vi "Get Log Settings.vi"(0 "Log Ref in":T2 format="%.0x", 7 "RT Data in":T1={"Device Ref"=18446744073709551615, "Waveforms"=[], "Channels"={"Command Chan Refs"=[], "Command Data Refs"=[], "Command Values"=[], "Status Chan Refs"=[], "Status Data Refs"=[], "Status Values"=[], "System Time"={"System Time"=timestamp(0 s since 1904-01-01), "Data Reference"=0, "Absolute Time Channel Data Ref"=0, "Get Date-Time Channel Data Ref"=0}, "Trigger Chan Refs"=[], "Trigger Data Refs"=[], "Trigger Values"=[]}, "Waveform Logs"=[], "Communication"={"Async Status"=refnum, "Wfm Comm Properties"={"WPL"={"Custom Queue Size"=1, "Use Custom Queue Size?"=FALSE}}, "Shutdown Event"=refnum, "Trigger Event"=refnum, "New File Event"=refnum, "Log Queues"=[], "Async VI Ref"=refnum}, "error"={"status"=FALSE, "code"=0, "source"=""}} {"Device Ref" format="%.0x"; "Channels"."Trigger Data Refs"."Data Reference" format="%.0x"; "Channels"."Trigger Chan Refs" format="%.0x"; "Channels"."System Time"."Get Date-Time Channel Data Ref" format="%.0x"; "Channels"."System Time"."Absolute Time Channel Data Ref" format="%.0x"; "Channels"."System Time"."Channel Data Reference" format="%.0x"; "Channels"."Status Data Refs"."Data Reference" format="%.0x"; "Channels"."Command Data Refs"."Data Reference" format="%.0x"; "Channels"."Status Chan Refs" format="%.0x"; "Channels"."Command Chan Refs" format="%.0x"; "Waveforms"."Waveform Ref in" format="%.0x"; "Waveform Logs"."Node ID" format="%.0x"; "Waveform Logs"."TDMS Error Code"."Data Ref" format="%.0x"; "Waveform Logs"."Missed Samples"."Data Ref" format="%.0x"; "Waveform Logs"."File Status"."Data Ref" format="%.0x"; "Waveform Logs"."Start New File"."Data Ref" format="%.0x"; "Waveform Logs"."Logging Enabled"."Data Ref" format="%.0x"; "Waveform Logs"."Stop Trigger"."Node Data Ref" format="%.0x"; "Waveform Logs"."Stop Trigger"."Node ID" format="%.0x"; "Waveform Logs"."Start Trigger"."Node Data Ref" format="%.0x"; "Waveform Logs"."Start Trigger"."Node ID" format="%.0x"}, 11 "Log Index in":i32) -> (8 "RT Data out":T1={"Device Ref"=18446744073709551615, "Waveforms"=[], "Channels"={"Command Chan Refs"=[], "Command Data Refs"=[], "Command Values"=[], "Status Chan Refs"=[], "Status Data Refs"=[], "Status Values"=[], "System Time"={"System Time"=timestamp(0 s since 1904-01-01), "Data Reference"=0, "Absolute Time Channel Data Ref"=0, "Get Date-Time Channel Data Ref"=0}, "Trigger Chan Refs"=[], "Trigger Data Refs"=[], "Trigger Values"=[]}, "Waveform Logs"=[], "Communication"={"Async Status"=refnum, "Wfm Comm Properties"={"WPL"={"Custom Queue Size"=1, "Use Custom Queue Size?"=FALSE}}, "Shutdown Event"=refnum, "Trigger Event"=refnum, "New File Event"=refnum, "Log Queues"=[], "Async VI Ref"=refnum}, "error"={"status"=FALSE, "code"=0, "source"=""}} {"Device Ref" format="%.0x"; "Channels"."Trigger Data Refs"."Data Reference" format="%.0x"; "Channels"."Trigger Chan Refs" format="%.0x"; "Channels"."System Time"."Get Date-Time Channel Data Ref" format="%.0x"; "Channels"."System Time"."Absolute Time Channel Data Ref" format="%.0x"; "Channels"."System Time"."Channel Data Reference" format="%.0x"; "Channels"."Status Data Refs"."Data Reference" format="%.0x"; "Channels"."Command Data Refs"."Data Reference" format="%.0x"; "Channels"."Status Chan Refs" format="%.0x"; "Channels"."Command Chan Refs" format="%.0x"; "Waveforms"."Waveform Ref in" format="%.0x"; "Waveform Logs"."Node ID" format="%.0x"; "Waveform Logs"."TDMS Error Code"."Data Ref" format="%.0x"; "Waveform Logs"."Missed Samples"."Data Ref" format="%.0x"; "Waveform Logs"."File Status"."Data Ref" format="%.0x"; "Waveform Logs"."Start New File"."Data Ref" format="%.0x"; "Waveform Logs"."Logging Enabled"."Data Ref" format="%.0x"; "Waveform Logs"."Stop Trigger"."Node Data Ref" format="%.0x"; "Waveform Logs"."Stop Trigger"."Node ID" format="%.0x"; "Waveform Logs"."Start Trigger"."Node Data Ref" format="%.0x"; "Waveform Logs"."Start Trigger"."Node ID" format="%.0x"}, 15 "Log Index out":i32)   [LabVIEW 2015, in "Waveform Data Logger Engine.lvlib"]
uses:
  Waveform Data Logger Engine.lvlib
  <vilib>/NI Veristand/Custom Device API/Custom Device Item Ref.ctl
  Types/RT Data.ctl
  Types/Inline Waveform Info.ctl
  <vilib>/NI Veristand/Custom Device API/Waveform Data Reference.ctl
  Classes/Waveforms/Waveform Receive/Associated Log.ctl
  <vilib>/NI Veristand/Custom Device API/Custom Device Waveform DataType.ctl
  Types/Channels.ctl
  <vilib>/NI Veristand/Custom Device API/Block Data Reference.ctl
  <vilib>/NI Veristand/Custom Device API/Data Reference.ctl
  Types/System Time.ctl
  Types/Inline Waveform Log Info.ctl
  Classes/Log File Specifications/Waveform TDMS Log File Specification/Waveform TDMS Log File Specification.lvclass
  Classes/Triggers/Trigger/Trigger.lvclass
  Types/Inline Log Waveform.ctl
  Types/Trigger Settings.ctl
  Types/Log Status.ctl
  Types/Channel.ctl
  Types/Communication.ctl
  Types/Async Status.ctl
  Types/Async State.ctl
  <vilib>/NI Veristand/Custom Device Waveform API/Communication Properties.ctl
  Types/Trigger Event Data.ctl
  Types/Trigger Received.ctl
  Types/New File Event Data.ctl
  Types/Log Queues.ctl
  Shared/Globals/Property Strings.vi
  Shared/Globals/Global GUIDs.vi
  <vilib>/NI Veristand/Custom Device API/Get Item Property (Boolean).vi
  <vilib>/NI Veristand/Custom Device API/Get Item Property (U16).vi
  <vilib>/NI Veristand/Custom Device API/Get Item Property (Double).vi
  <vilib>/NI Veristand/Custom Device API/Custom Device API.lvlib
  Shared/Waveform Data Logger Shared.lvlib
  Classes/Waveforms/Waveform Receive/Waveform Receive.lvclass
  <vilib>/NI Veristand/Custom Device Waveform API/NI_VS Custom Device Waveform API.lvlib
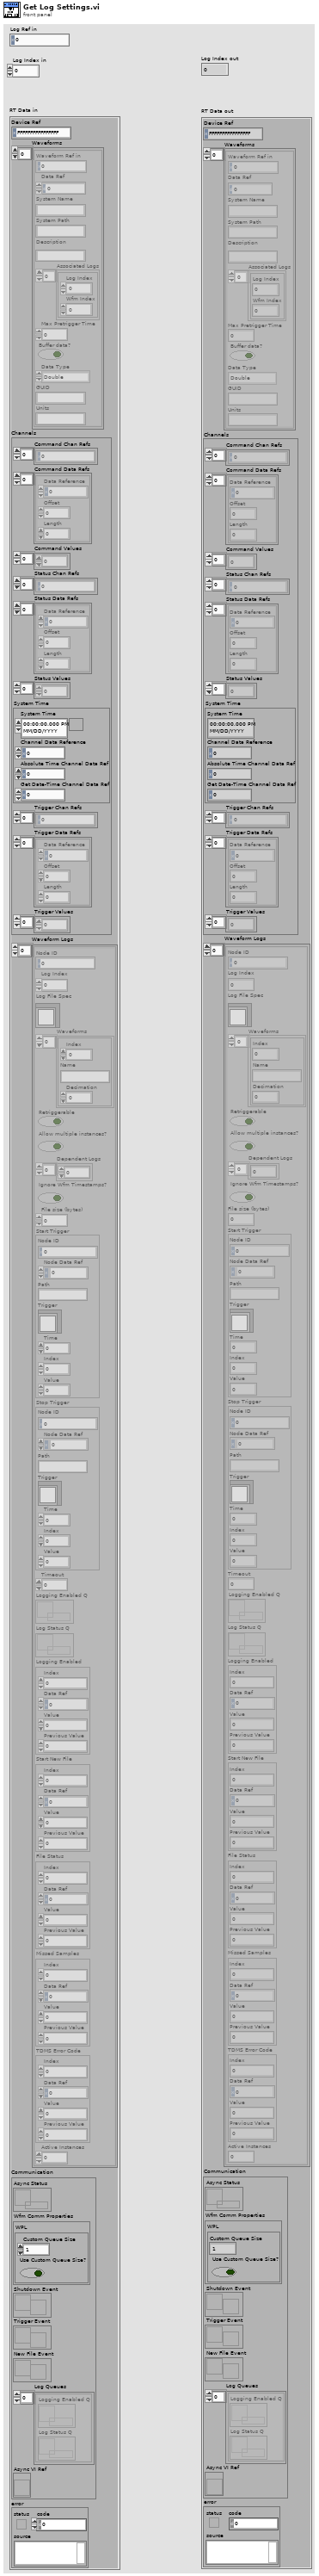
[diagram p1: front panel]
types:
  T1 = typedef "Waveform Data Logger Engine.lvlib/RT Data.ctl" = cluster{"Device Ref":T2, "Waveforms":T3[], "Channels":T7, "Waveform Logs":T11[], "Communication":T15, "error":errorcluster}
  T2 = typedef "Custom Device API.lvlib/Custom Device Item Ref.ctl" = u64
  T3 = typedef "Waveform Data Logger Engine.lvlib/Inline Waveform Info.ctl" = cluster{"Waveform Ref in":T2, "Data Ref":T4, "System Name":string, "System Path":string, "Description":string, "Associated Logs":T5[], "Max Pretrigger Time":dbl, "Buffer data?":bool, "Data Type":T6, "GUID":string, "Units":string}
  T4 = typedef "Custom Device API.lvlib/Waveform Data Reference.ctl" = i32
  T5 = typedef "Waveform Receive.lvclass/Associated Log.ctl" = cluster{"Log Index":i32, "Wfm Index":i32}
  T6 = typedef "Custom Device API.lvlib/Custom Device Waveform DataType.ctl" = enum16{"Double", "Complex Double"}
  T7 = typedef "Waveform Data Logger Engine.lvlib/Channels.ctl" = cluster{"Command Chan Refs":T2[], "Command Data Refs":T8[], "Command Values":dbl[], "Status Chan Refs":T2[], "Status Data Refs":T8[], "Status Values":dbl[], "System Time":T10, "Trigger Chan Refs":T2[], "Trigger Data Refs":T8[], "Trigger Values":dbl[]}
  T8 = typedef "Custom Device API.lvlib/Block Data Reference.ctl" = cluster{"Data Reference":T9, "Offset":u64, "Length":u64}
  T9 = typedef "Custom Device API.lvlib/Data Reference.ctl" = i32
  T10 = typedef "Waveform Data Logger Engine.lvlib/System Time.ctl" = cluster{"System Time":timestamp, "Data Reference":T9, "Absolute Time Channel Data Ref":T9, "Get Date-Time Channel Data Ref":T9}
  T11 = typedef "Waveform Data Logger Engine.lvlib/Inline Waveform Log Info.ctl" = cluster{"Node ID":T2, "Log Index":i32, "Log File Spec":refnum<class "Waveform TDMS Log File Specification.lvclass">, "Waveforms":T12[], "Retriggerable":bool, "Allow multiple instances?":bool, "Dependent Logs":i32[], "Ignore Wfm Timestamps?":bool, "File size (bytes)":i64, "Start Trigger":T13, "Stop Trigger":T13, "Timeout":dbl, "Logging Enabled Q":refnum<queue>, "Log Status Q":refnum<queue>, "Logging Enabled":T14, "Start New File":T14, "File Status":T14, "Missed Samples":T14, "TDMS Error Code":T14, "Active Instances":i32}
  T12 = typedef "Waveform Data Logger Engine.lvlib/Inline Log Waveform.ctl" = cluster{"Index":i32, "Name":string, "Decimation":u32}
  T13 = typedef "Waveform Data Logger Engine.lvlib/Trigger Settings.ctl" = cluster{"Node ID":T2, "Node Data Ref":i32, "Path":string, "Trigger":refnum<class "Trigger.lvclass">, "Time":dbl, "Index":i32, "Value":dbl}
  T14 = typedef "Waveform Data Logger Engine.lvlib/Channel.ctl" = cluster{"Index":i32, "Data Ref":T9, "Value":dbl, "Previous Value":dbl}
  T15 = typedef "Waveform Data Logger Engine.lvlib/Communication.ctl" = cluster{"Async Status":refnum<queue>, "Wfm Comm Properties":T16, "Shutdown Event":refnum<user-event>, "Trigger Event":refnum<user-event>, "New File Event":refnum<user-event>, "Log Queues":T17[], "Async VI Ref":refnum<vi>}
  T16 = typedef "NI_VS Custom Device Waveform API.lvlib/Communication Properties.ctl" = cluster{"WPL":cluster{"Custom Queue Size":i32, "Use Custom Queue Size?":bool}}
  T17 = typedef "Waveform Data Logger Engine.lvlib/Log Queues.ctl" = cluster{"Logging Enabled Q":refnum<queue>, "Log Status Q":refnum<queue>}
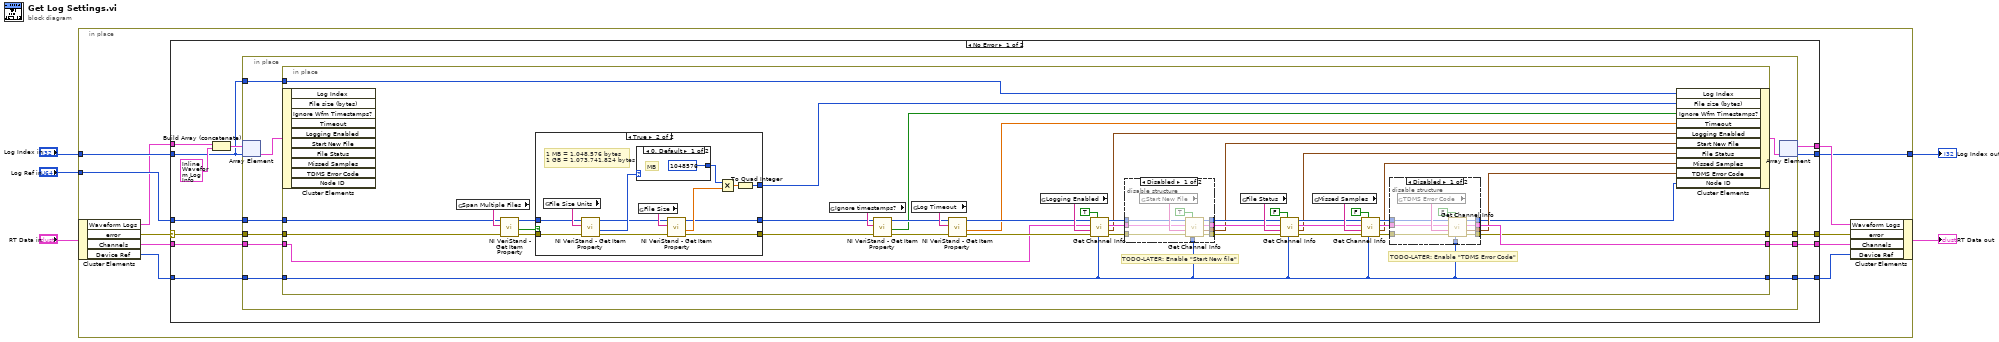
[diagram p0: block diagram]
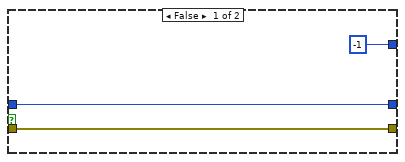
[diagram p4: hidden frame]
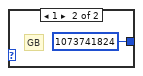
[diagram p5: hidden frame]
diagram:
  n1 = in-place {
    in-place-border: "Log Index in" -> [w16]
    in-place-border: "Log Ref in" -> [w13]
    in-place-border: [w10] -> w1
    n2 = in-place-cluster #1("RT Data in") -> ("Waveform Logs"=w12:T11[], "error"=w15:errorcluster, "Channels"=w7:T7, "Device Ref"=w8:T2)
    n3 = case shown="No Error" w15 {
      selector: w15 -> [w28 w134]
      tunnel: [w26 w134] -> w14
      tunnel: w13 -> [w29 _]
      tunnel: w16 -> [w21 w130]
      tunnel: w7 -> [w27 w133]
      tunnel: [w25 w133] -> w6
      tunnel: w8 -> [w18 w132]
      tunnel: [w17 w132] -> w9
      tunnel: w12 -> [w24 w131]
      tunnel: [w20 w131] -> w11
      tunnel: [w19 w130] -> w10
      frame No Error {
        n4 = Build Array (concatenate)(w24, T11 {"Node ID"=0, "Log Index"=0, "Log File Spec"=refnum, "Waveforms"=[], "Retriggerable"=FALSE, "Allow multiple instances?"=FALSE, "Dependent Logs"=[], "Ignore Wfm Timestamps?"=FALSE, "File size (bytes)"=0, "Start Trigger"={"Node ID"=0, "Node Data Ref"=0, "Path"="", "Trigger"=refnum, "Time"=0.0, "Index"=0, "Value"=0.0}, "Stop Trigger"={"Node ID"=0, "Node Data Ref"=0, "Path"="", "Trigger"=refnum, "Time"=0.0, "Index"=0, "Value"=0.0}, "Timeout"=0.0, "Logging Enabled Q"=refnum, "Log Status Q"=refnum, "Logging Enabled"={"Index"=0, "Data Ref"=0, "Value"=0.0, "Previous Value"=0.0}, "Start New File"={"Index"=0, "Data Ref"=0, "Value"=0.0, "Previous Value"=0.0}, "File Status"={"Index"=0, "Data Ref"=0, "Value"=0.0, "Previous Value"=0.0}, "Missed Samples"={"Index"=0, "Data Ref"=0, "Value"=0.0, "Previous Value"=0.0}, "TDMS Error Code"={"Index"=0, "Data Ref"=0, "Value"=0.0, "Previous Value"=0.0}, "Active Instances"=0} ("Waveform Log in")) -> (w22:T11[])
        n5 = in-place {
          in-place-border: w29 -> [w39]
          in-place-border: w28 -> [w38]
          in-place-border: w21 -> [w37]
          in-place-border: w27 -> [w36]
          in-place-border: [w35] -> w26
          in-place-border: [w34] -> w25
          in-place-border: w18 -> [w33]
          in-place-border: [w30] -> w17
          n6 = in-place-array #2(w22, w21) -> (w32:T11)
          n7 = in-place {
            in-place-border: w39 -> [w80]
            in-place-border: w38 -> [w79]
            in-place-border: w37 -> [w43]
            in-place-border: w36 -> [w70]
            in-place-border: [w41] -> w35
            in-place-border: [w54] -> w34
            in-place-border: w33 -> [w42]
            in-place-border: [w42] -> w30
            # "TODO-LATER: Enable \"TDMS Error Code\""
            # "TODO-LATER: Enable \"Start New file\""
            n8 = in-place-cluster #3(w32) -> ()  [unwired: 10 out]
            n9 = global read "Property Strings.vi" "Span Multiple Files"() -> (w84:string)
            n10 = call-poly <vilib>:"NI VeriStand - Get Item Property.vi"("error in (no error)"=w79, "Property Name"=w84, "Item Ref in"=w80) -> ("error out"=w82:errorcluster, "Value"=w83:bool, "Item Ref out"=w81:T2)  [unwired: 1 in, 5 out]
            n11 = case shown="True" w83 {
              tunnel: w82 -> [w112 w119]
              tunnel: w81 -> [w113 w120]
              tunnel: [i64 -1 ("File size (bytes)") w123] -> w44
              tunnel: [w113 w116] -> w78
              tunnel: [w112 w115] -> w77
              frame False {
              }
              frame True {
                # "1 MB = 1,048,576 bytes\n1 GB = 1,073,741,824 bytes"
                n12 = global read "Property Strings.vi" "File Size Units"() -> (w126:string)
                n13 = call-poly <vilib>:"NI VeriStand - Get Item Property.vi"("error in (no error)"=w119, "Property Name"=w126, "Item Ref in"=w120) -> ("error out"=w117:errorcluster, "Value"=w121:u16, "Item Ref out"=w118:T2)  [unwired: 1 in, 5 out]
                n14 = case shown="0, Default" w121 {
                  tunnel: [1048576 1073741824] -> w124
                  frame 0, Default {
                    # "MB"
                  }
                  frame 1 {
                    # "GB"
                  }
                }
                n15 = global read "Property Strings.vi" "File Size"() -> (w127:string)
                n16 = call-poly <vilib>:"NI VeriStand - Get Item Property.vi"("error in (no error)"=w117, "Property Name"=w127, "Item Ref in"=w118) -> ("error out"=w115:errorcluster, "Value"=w125:dbl, "Item Ref out"=w116:T2)  [unwired: 1 in, 5 out]
                n17 = Multiply(x=w124, y=w125) -> (x*y=w122:dbl)
                n18 = To Quad Integer(1:w122) -> (0:w123:i64)
              }
            }
            n19 = global read "Property Strings.vi" "Ignore timestamps?"() -> (w85:string)
            n20 = call-poly <vilib>:"NI VeriStand - Get Item Property.vi"("error in (no error)"=w77, "Property Name"=w85, "Item Ref in"=w78) -> ("error out"=w74:errorcluster, "Value"=w45:bool, "Item Ref out"=w75:T2)  [unwired: 1 in, 5 out]
            n21 = global read "Property Strings.vi" "Log Timeout"() -> (w76:string)
            n22 = call-poly <vilib>:"NI VeriStand - Get Item Property.vi"("error in (no error)"=w74, "Property Name"=w76, "Item Ref in"=w75) -> ("error out"=w73:errorcluster, "Value"=w46:dbl, "Item Ref out"=w53:T2)  [unwired: 1 in, 5 out]
            n23 = global read "Global GUIDs.vi" "Logging Enabled"() -> (w72:string)
            n24 = call "Get Channel Info.vi"("Device Ref in"=w42, "Command?"=TRUE, "error in (no error)"=w73, "Item GUID"=w72, "Channel Refs in"=w70, "Item Ref in"=w53) -> ("error out"=w68:errorcluster, "Channel out"=w47:T14, "Channel Refs out"=w69:T7, "Item Ref out"=w52:T2)  [unwired: 2 in]
            n25 = disable-structure shown="Disabled" {
              disable-tunnel: w52 -> [w106 w109]
              disable-tunnel: w69 -> [w105 w111]
              disable-tunnel: w68 -> [w104 w110]
              disable-tunnel: [w103 _] -> w48
              disable-tunnel: [w102 w109] -> w63
              disable-tunnel: [w101 w111] -> w60
              disable-tunnel: [w100 w110] -> w59
              disable-tunnel: w42 -> [w99 _]
              frame Disabled {
                n26 = global read "Global GUIDs.vi" "Start New File"() -> (w107:string)
                n27 = call "Get Channel Info.vi"("Device Ref in"=w99, "Command?"=TRUE, "error in (no error)"=w104, "Item GUID"=w107, "Channel Refs in"=w105, "Item Ref in"=w106) -> ("error out"=w100:errorcluster, "Channel out"=w103:T14, "Channel Refs out"=w101:T7, "Item Ref out"=w102:T2)  [unwired: 2 in]
              }
              frame Enabled {
              }
            }
            n28 = global read "Global GUIDs.vi" "File Status"() -> (w67:string)
            n29 = call "Get Channel Info.vi"("Device Ref in"=w42, "Command?"=FALSE, "error in (no error)"=w59, "Item GUID"=w67, "Channel Refs in"=w60, "Item Ref in"=w63) -> ("error out"=w58:errorcluster, "Channel out"=w49:T14, "Channel Refs out"=w61:T7, "Item Ref out"=w62:T2)  [unwired: 2 in]
            n30 = global read "Global GUIDs.vi" "Missed Samples"() -> (w64:string)
            n31 = call "Get Channel Info.vi"("Device Ref in"=w42, "Command?"=FALSE, "error in (no error)"=w58, "Item GUID"=w64, "Channel Refs in"=w61, "Item Ref in"=w62) -> ("error out"=w55:errorcluster, "Channel out"=w50:T14, "Channel Refs out"=w56:T7, "Item Ref out"=w57:T2)  [unwired: 2 in]
            n32 = disable-structure shown="Disabled" {
              disable-tunnel: w57 -> [w93 w96]
              disable-tunnel: w56 -> [w92 w98]
              disable-tunnel: w55 -> [w91 w97]
              disable-tunnel: [w90 w97] -> w41
              disable-tunnel: [w89 w98] -> w54
              disable-tunnel: [w88 _] -> w51
              disable-tunnel: w42 -> [w87 _]
              disable-tunnel: [w86 w96] -> w40
              frame Disabled {
                n33 = global read "Global GUIDs.vi" "TDMS Error Code"() -> (w95:string)
                n34 = call "Get Channel Info.vi"("Device Ref in"=w87, "Command?"=FALSE, "error in (no error)"=w91, "Item GUID"=w95, "Channel Refs in"=w92, "Item Ref in"=w93) -> ("error out"=w90:errorcluster, "Channel out"=w88:T14, "Channel Refs out"=w89:T7, "Item Ref out"=w86:T2)  [unwired: 2 in]
              }
              frame Enabled {
              }
            }
            n35 = in-place-cluster #3("Log Index"=w43, "File size (bytes)"=w44, "Ignore Wfm Timestamps?"=w45, "Timeout"=w46, "Logging Enabled"=w47, "Start New File"=w48, "File Status"=w49, "Missed Samples"=w50, "TDMS Error Code"=w51, "Node ID"=w40) -> (w31:T11)
          }
          n36 = in-place-array #2(w31) -> (w20:T11[], w19:i32)
        }
      }
      frame Error {
      }
    }
    n37 = in-place-cluster #1("Waveform Logs"=w11, "error"=w14, "Channels"=w6, "Device Ref"=w9) -> (→"RT Data out":T1)
  }
  "Log Index out" <- w1
